vi "oopAPI_TX (Generic)_2.vi"() -> ()   [LabVIEW 2020]
uses:
  src/_controls/queue_data_full.ctl
  src/_controls/queue_header_generic.ctl
  src/_polimorphicInstances/session/Fdx Create Session (Tx-Generic).vi
  src/_polimorphicInstances/session/Fdx Close Session (Port).vi
  src/AIM664LV.lvlib
  src/helpers/EthFrameManagement/EthFrameManagement.lvlib
panel:
  in  "PortMap":u32
  out "Duplicated":bool
  in  "size":i32=100
  out "x-y":u32(graph)=1
  in  "HeaderInfo":T1={"InterFrameGap"=25, "PacketGroupWaitTime"=5000, "PayloadBufferMode"=0, "PayloadGenerationMode"=0, "PreambleCount"=7, "Skew"=0, "NetSelect"=3, "FrameStartMode"=1, "PhysErrorInjection"=0, "SequenceNumberInit"=65535, "SequenceNumberOffset"=65535} {"NetSelect" items=["FDX_TX_FRAME_DLY_A"=0, "FDX_TX_FRAME_DLY_B"=1, "FDX_TX_FRAME_BOTH "=3, "FDX_TX_FRAME_ONLY_A"=4, "FDX_TX_FRAME_ONLY_B "=5]; "FrameStartMode" items=["FDX_TX_FRAME_START_IFG", "FDX_TX_FRAME_START_PGWT", "FDX_TX_FRAME_START_TRG"]; "PhysErrorInjection" items=["FDX_TX_FRAME_ERR_OFF"=0, "FDX_TX_FRAME_ERR_CRC"=1, "FDX_TX_FRAME_ERR_ALI"=2, "FDX_TX_FRAME_ERR_PRE"=4, "FDX_TX_FRAME_ERR_PHY"=8]; "SequenceNumberInit" items=["FDX_TX_FRAME_SEQ_INIT_AUTO"=65535]; "SequenceNumberOffset" items=["FDX_TX_FRAME_SEQ_OFFS_AUTO "=65535]; "PayloadGenerationMode" items=["FDX_TX_FRAME_PGM_USER"=0, "FDX_TX_FRAME_PGM_IP_PART"=1, "FDX_TX_FRAME_PGM_IP_FULL"=2, "FDX_TX_FRAME_PGM_IP_PART_TT"=10, "FDX_TX_FRAME_PGM_IP_FULL_TT"=20]; "PayloadBufferMode" items=["FDX_TX_FRAME_PBM_STD", "FDX_TX_FRAME_PBM_MAC", "FDX_TX_FRAME_PBM_UDP"]}
  in  "VL Id":u16=60
  in  "configuration":T2={"domainID"=1, "sideID"=1, "locationID"=1, "interfaceID"=1, "partitionID"=1} {"interfaceID" format="%.0b"}
  out "Payload":u8[](array[numeric]) format="%.0x"
  in  "UDPdstPort":u16=1
  in  "UDPsrcPort":u16=1
  out "TxStatus":T3={"TxStatus"=1, "Frames"=855, "TransmitMode"=0, "FramesPortB"=0}
  out "TxQueueStatus":T4={"QueueStatus"=0, "BytesReloadable"=0, "FramesSent"=854, "FramesInCycQueue"=0} {"QueueStatus" items=["FDX_QUE_EMPTY", "FDX_QUE_FILLED", "FDX_QUE_FULL", "FDX_QUE_SENT", "FDX_QUE_CYCL_RUN", "FDX_QUE_CYCL_SENT"]}
  out "TxQueueInfo":cluster{"QueueBaseAddr":u32, "QueueSizeOut":u32}={"QueueBaseAddr"=50892800, "QueueSizeOut"=4194304}
  out "QueueSizeIn":u32
  in  "port":u32
  in  "board":u32
  out "current time":timestamp=timestamp(3686777794.875688 s since 1904-01-01)
  out "current irig time":T5={"SignOut"=40, "DayOut"=303, "HourOut"=0, "MinOut"=56, "SecondOut"=34, "MilliSecOut"=727, "MicroSecOut"=281, "NanoSecOut"=400, "InfoOut"=0, "Mode"=3}
  in  "stop":bool
  out "PortInitOut":T6={"PortConfig"=0, "PortUsed"=1, "GlobalMemFree"=0, "SharedMemFree"=0} {"PortConfig" items=["FDX_SINGLE", "FDX_REDUNDANT"]}
  out "error out":errorcluster
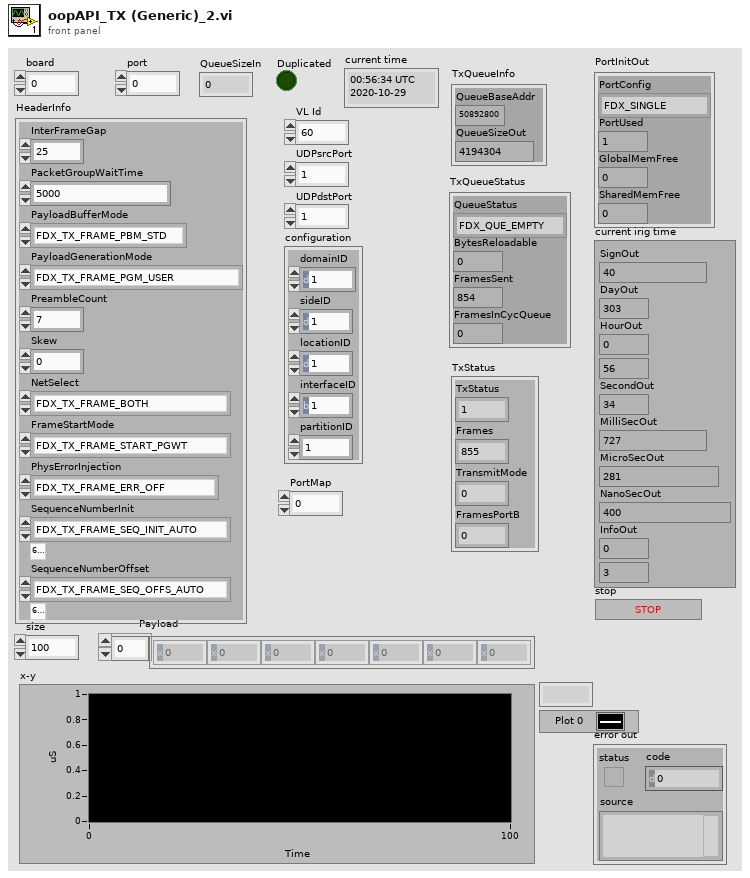
[diagram p1: front panel]
types:
  T1 = typedef "AIM664LV.lvlib/queue_header_generic.ctl" = cluster{"InterFrameGap":u32, "PacketGroupWaitTime":u32, "PayloadBufferMode":u8, "PayloadGenerationMode":u8, "PreambleCount":u8, "Skew":u32, "NetSelect":u8, "FrameStartMode":u8, "PhysErrorInjection":u32, "SequenceNumberInit":u16, "SequenceNumberOffset":u16}
  T2 = typedef "AIM664LV.lvlib/queue_data_full.ctl" = cluster{"domainID":u8, "sideID":u8, "locationID":u8, "interfaceID":u8, "partitionID":u8}
  T3 = cluster{"TxStatus":u32, "Frames":u32, "TransmitMode":u32, "FramesPortB":u32}
  T4 = cluster{"QueueStatus":i32, "BytesReloadable":u32, "FramesSent":u32, "FramesInCycQueue":u32}
  T5 = cluster{"SignOut":i32, "DayOut":u32, "HourOut":u32, "MinOut":u32, "SecondOut":u32, "MilliSecOut":u32, "MicroSecOut":u32, "NanoSecOut":u32, "InfoOut":u32, "Mode":u32}
  T6 = cluster{"PortConfig":u32, "PortUsed":u32, "GlobalMemFree":u32, "SharedMemFree":u32}
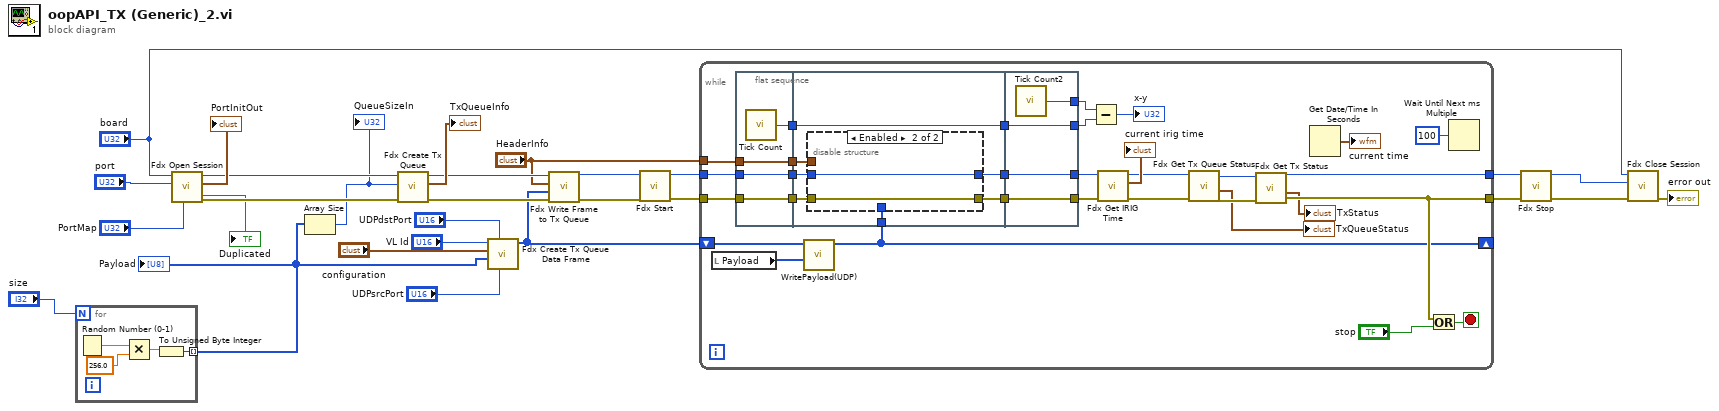
[diagram p0: block diagram]
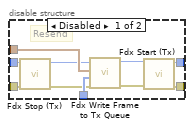
[diagram p2: hidden frame]
diagram:
  n1 = for {
    N: "size" -> [_]
    tunnel: [w29] -> w5 mode=indexing
    n2 = Random Number (0-1)() -> (number: 0 to 1=w32:dbl)
    n3 = Multiply(x=w32, y=256.0) -> (x*y=w30:dbl)
    n4 = To Unsigned Byte Integer(number=w30) -> (unsigned 8bit integer=w29:u8)
  }
  "Payload" <- w5
  n5 = call-poly "Fdx Open Session.vi"("PortMap"="PortMap", "port"="port", "board"="board") -> ("error out"=w21:errorcluster, "PortInitOut"=→"PortInitOut":T6, "port handle out"=w22:u32, "Duplicated"=→"Duplicated":bool)  [unwired: 4 in, 1 out]
  n6 = Array Size(array=w5) -> (size(s)=w7:i32)
  "QueueSizeIn" <- w7
  n7 = call "Fdx Create Tx Queue.vi"("error in (no error)"=w21, "QueueSizeIn"=w7, "InstrumentHandle_port in"=w22) -> ("error out"=w19:errorcluster, "TxQueueInfo"=→"TxQueueInfo":cluster{"QueueBaseAddr":u32, "QueueSizeOut":u32}, "InstrumentHandle_port out"=w16:u32)  [unwired: 6 in]
  n8 = call "Fdx Create Tx Queue Data Frame.vi"("UDPsrcPort"="UDPsrcPort", "UDPdstPort"="UDPdstPort", "Payload"=w5, "afdx configuration"="configuration", "VL Id"="VL Id") -> ("Frame"=w9:u8[])  [unwired: 6 in]
  n9 = call "Fdx Write Frame to Tx Queue.vi"("error in (no error)"=w19, "Frame in"=w9, "HeaderInfo"="HeaderInfo", "InstrumentHandle_port in"=w16) -> ("error out"=w18:errorcluster, "InstrumentHandle_port out"=w17:u32)  [unwired: 6 in]
  n10 = call-poly "Fdx Start.vi"("error in (no error)"=w18, "InstrumentHandle_port in"=w17) -> ("error out"=w26:errorcluster, "InstrumentHandle_port out"=w25:u32)  [unwired: 8 in]
  n11 = while {
    tunnel: w26 -> [w45]
    tunnel: w25 -> [w46]
    tunnel: [w54] -> w15
    tunnel: [w53] -> w14
    shift-right: [w48] -> _
    shift-left: w9 -> [w50]
    tunnel: "HeaderInfo" -> [w49]
    stop <- w62 stop-if-true
    n12 = local read "Payload"() -> (w47:u8[])
    n13 = flat-sequence {
      tunnel: w45 -> [w65]
      tunnel: w46 -> [w66]
      tunnel: w49 -> [w67]
      tunnel: [w67] -> w42
      tunnel: [w66] -> w41
      tunnel: [w65] -> w40
      tunnel: [w64] -> w37
      tunnel: w48 -> [w73]
      tunnel: w42 -> [w74]
      tunnel: w41 -> [w72]
      tunnel: w40 -> [w71]
      tunnel: [w70] -> w39
      tunnel: [w69] -> w38
      tunnel: w37 -> [w68]
      tunnel: [w68] -> w36
      tunnel: [w89] -> w43
      tunnel: [w90] -> w44
      tunnel: w39 -> [w90]
      tunnel: w38 -> [w89]
      tunnel: w36 -> [w88]
      tunnel: [w88] -> w34
      tunnel: [w87] -> w35
      frame #0 {
        n14 = call "Tick Count"() -> ("Tick Count(uSec)"=w64:u32)
      }
      frame #1 {
        n15 = disable-structure shown="Enabled" {
          disable-tunnel: w74 -> [w84 _]
          disable-tunnel: w73 -> [w83 _]
          disable-tunnel: w72 -> [w82 w85]
          disable-tunnel: w71 -> [w81 w86]
          disable-tunnel: [w80 w86] -> w70
          disable-tunnel: [w79 w85] -> w69
          frame Disabled {
            # "Resend"
            n16 = call "Fdx Stop (Tx).vi"("error in (no error)"=w81, "InstrumentHandle_port in"=w82) -> ("error out"=w77:errorcluster, "InstrumentHandle_port out"=w78:u32)  [unwired: 8 in]
            n17 = call "Fdx Write Frame to Tx Queue.vi"("error in (no error)"=w77, "Frame in"=w83, "HeaderInfo"=w84, "InstrumentHandle_port in"=w78) -> ("error out"=w75:errorcluster, "InstrumentHandle_port out"=w76:u32)  [unwired: 6 in]
            n18 = call "Fdx Start (Tx).vi"("error in (no error)"=w75, "InstrumentHandle_port in"=w76) -> ("error out"=w80:errorcluster, "InstrumentHandle_port out"=w79:u32)  [unwired: 8 in]
          }
          frame Enabled {
          }
        }
      }
      frame #2 {
        n19 = call "Tick Count2"() -> ("Tick Count(uSec)"=w87:u32)
      }
    }
    n20 = call "WritePayload(UDP).vi"("Payload"=w47, "Ethernet Frame In"=w50) -> ("Ethernet Frame Out"=w48:u8[])  [unwired: 9 in]
    n21 = Subtract(x=w35, y=w34) -> (x-y=→"x-y":u32)
    n22 = call "Fdx Get IRIG Time.vi"("error in (no error)"=w44, "InstrumentHandle_board in"=w43) -> ("error out"=w57:errorcluster, "Curent Irig Time"=→"current irig time":T5, "InstrumentHandle_board out"=w58:u32)  [unwired: 7 in]
    n23 = call "Fdx Get Tx Queue Status.vi"("error in (no error)"=w57, "InstrumentHandle in"=w58) -> ("error out"=w55:errorcluster, "TxQueueStatus"=→"TxQueueStatus":T4, "InstrumentHandle out"=w56:u32)  [unwired: 7 in]
    n24 = call "Fdx Get Tx Status.vi"("error in (no error)"=w55, "InstrumentHandle_port in"=w56) -> ("error out"=w54:errorcluster, "TxStatus"=→"TxStatus":T3, "InstrumentHandle_port out"=w53:u32)  [unwired: 7 in]
    n25 = Get Date/Time In Seconds() -> (seconds since 1Jan1904=→"current time":timestamp)
    n26 = Or(x=w54, y="stop") -> (x .or. y?=w62:bool)
    n27 = Wait Until Next ms Multiple(millisecond multiple=u32 100) -> ()  [unwired: 1 out]
  }
  n28 = call-poly "Fdx Stop.vi"("error in (no error)"=w15, "InstrumentHandle_port in"=w14) -> ("error out"=w23:errorcluster, "InstrumentHandle_port out"=w2:u32)  [unwired: 8 in]
  n29 = call-poly "Fdx Close Session.vi"("error in"=w23, "InstrumentHandle_port in"=w2, "InstrumentHandle_board in"="board") -> ("error out"=→"error out":errorcluster)  [unwired: 8 in]
